vi "Convert to payload.vi"(8 "error in":errorcluster, 11 "Data":string[][](array[string])) -> (0 "error out":errorcluster, 3 "U8 Array":u8[](array[numeric]))   [LabVIEW 2025, in "CAN-LIN Raw Bus Capture.lvclass"]
uses:
  CAN-LIN Raw Bus Capture.lvclass
  CAN-LIN Raw Bus Capture.lvclass/CAN-LIN Raw Bus Capture.ctl
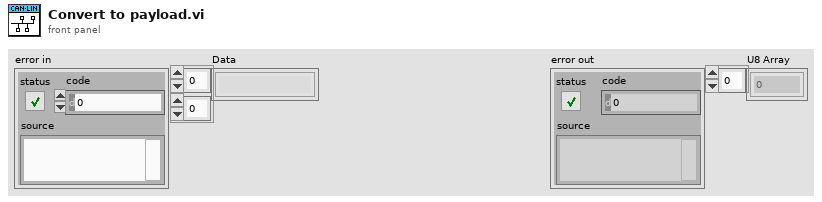
[diagram p1: front panel]
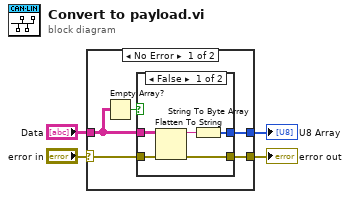
[diagram p0: block diagram]
diagram:
  n1 = case shown="No Error" "error in" {
    selector: "error in" -> [w9 w16]
    tunnel: [w8 w16] -> w3
    tunnel: [w7 _] -> w2
    tunnel: "Data" -> [w5 _]
    frame No Error {
      n2 = Empty Array?(array=w5) -> (empty?=w6:bool)
      n3 = case shown="False" w6 {
        tunnel: w9 -> [w14 w15]
        tunnel: [w13 w15] -> w8
        tunnel: [w10 _] -> w7
        tunnel: w5 -> [w12 _]
        frame False {
          n4 = Flatten To String(anything=w12, error in (no error)=w14) -> (data string=w11:string, error out=w13:errorcluster)  [unwired: 2 in, 1 out]
          n5 = String To Byte Array(string=w11) -> (unsigned byte array=w10:u8[])
        }
        frame True {
        }
      }
    }
    frame Error {
    }
  }
  "error out" <- w3
  "U8 Array" <- w2
